vi "RemovTeStatisticals.vi"(8 "error in (no error)":errorcluster caption="错误输入（无错误）", 11 "configuration file path":path caption="配置文件的路径") -> (0 "error out":errorcluster caption="错误输出", 3 "configuration file path 2":path caption="配置文件的路径")   [LabVIEW 2018]
uses:
  <vilib>/Utility/config.llb/Write Key (String).vi
  <vilib>/Utility/config.llb/NI_LVConfig.lvlib
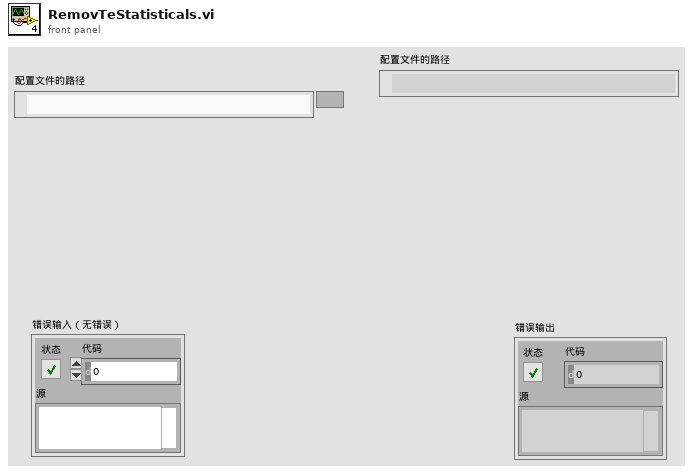
[diagram p1: front panel]
types:
  T1 = typedef "NI_LVConfig.lvlib/Config Data RefNum.ctl" = refnum<k1>
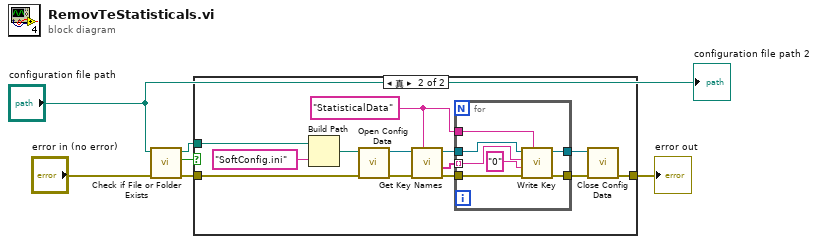
[diagram p0: block diagram]
diagram:
  n1 = call <vilib>:"Check if File or Folder Exists.vi"("error in (no error)"="error in (no error)", "path"="configuration file path") -> ("error out"=w2:errorcluster, "file or folder exists?"=w5:bool, "dup path"=w6:path)  [unwired: 7 in]
  n2 = case shown="真" w5 {
    tunnel: w6 -> [_ w18]
    tunnel: w2 -> [w7 w10]
    tunnel: [w7 w8] -> w1
    frame False {
    }
    frame True {
      w14 = "StatisticalData" ("section")
      n3 = Build Path(base path=w18, name or relative path="SoftConfig.ini" ("名称或相对路径")) -> (appended path=w20:path)
      n4 = call <vilib>:"Open Config Data.vi"("error in (no error)"=w10, "configuration file path"=w20) -> ("error out"=w9:errorcluster, "refnum"=w17:T1)  [unwired: 7 in, 1 out]
      n5 = call <vilib>:"Get Key Names.vi"("section"=w14, "error in (no error)"=w9, "refnum"=w17) -> ("error out"=w11:errorcluster, "key names"=w15:string[], "refnum out"=w16:T1)  [unwired: 5 in, 1 out]
      n6 = for {
        tunnel: w16 -> [w27]
        tunnel: w15 -> [w25] mode=indexing
        tunnel: w14 -> [w24]
        tunnel: [w23] -> w13
        tunnel: [w22] -> w12
        tunnel: w11 -> [w21]
        n7 = call-poly <vilib>:"Write Key.vi"("section"=w24, "error in (no error)"=w21, "value"="0" ("key"), "key"=w25, "refnum"=w27) -> ("error out"=w22:errorcluster, "refnum out"=w23:T1)  [unwired: 4 in, 1 out]
      }
      n8 = call <vilib>:"Close Config Data.vi"("error in (no error)"=w12, "refnum"=w13) -> ("error out"=w8:errorcluster)  [unwired: 8 in, 1 out]
    }
  }
  "error out" <- w1
  "configuration file path 2" <- "configuration file path"
